vi "Configure Multi Eval Meas Timeout.vi"(8 "error in (no error)":errorcluster, 9 "Measurement Timeout (0)":dbl format="%^.3e", 10 "Instance (1)":i32=1, 11 "VISA resource name":refnum<visa-resource-name>) -> (0 "error out":errorcluster, 3 "VISA resource name out":refnum<visa-resource-name>)   [LabVIEW 2020, in "Rohde&Schwarz CMP LR WPAN Measurement.lvlib"]
doc: "Defines a timeout for the measurement. The timer is started when the measurement is initiated via a READ or INIT command. It is not started if the measurement is initiated manually. When the measurement has completed the first measurement cycle (first single shot), the statistical depth is reached and the timer is reset. If the first measurement cycle has not been completed when the timer expires, the measurement is stopped. The measurement state changes to RDY. The reliability indicator is set to 1, indicating that a measurement timeout occurred. Still running READ, FETCh or CALCulate commands are completed, returning the available results. At least for some results, there are no values at all or the statistical depth has not been reached.\nA timeout of 0 s corresponds to an infinite measurement timeout.\n\nAttribute:\nRSCMPLRWM_ATTR_MULTIEVAL_TIMEOUT\n\nRemote-control command:\nCONFigure:WPAN:MEAS<i>:MEValuation:TOUT"
uses:
  <instrlib>/Rohde&Schwarz CMP LR WPAN Measurement/Rohde&Schwarz CMP LR WPAN Measurement.lvlib
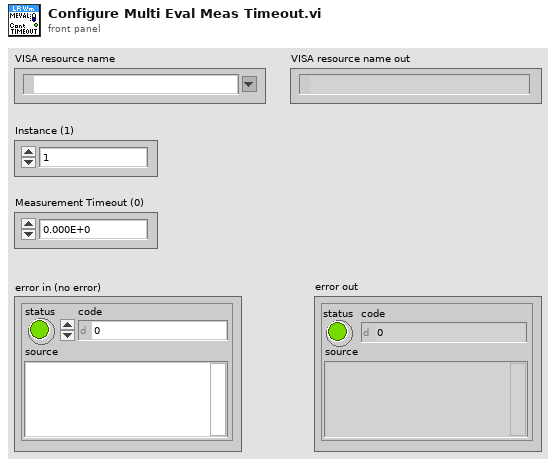
[diagram p1: front panel]
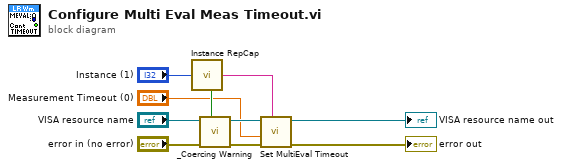
[diagram p0: block diagram]
diagram:
  n1 = call <instrlib>:"Instance RepCap.vi"("Instance In"="Instance (1)") -> ("In Range?"=w7:bool, "RepCap Identifier Out"=w8:string)  [unwired: 1 in]
  n2 = call <instrlib>:"_Coercing Warning.vi"("In Range?"=w7, "error in (no error)"="error in (no error)", "VISA resource name"="VISA resource name") -> ("error out"=w4:errorcluster, "VISA resource name out"=w3:refnum<visa-resource-name>)  [unwired: 7 in]
  n3 = call "Set MultiEval Timeout"("Repeated Capabilities"=w8, "error in (no error)"=w4, "MultiEval Timeout (0.0)"="Measurement Timeout (0)", "instrument handle"=w3) -> ("error out"=→"error out":errorcluster, "instrument handle out"=→"VISA resource name out":refnum<visa-resource-name>)  [unwired: 6 in]
